vi "createEvent.vi"(8 "error in (no error)":errorcluster, 11 "Event in":refnum<class "Event.lvclass">) -> (0 "error out":errorcluster, 3 "Event out":refnum<class "Event.lvclass">)   [LabVIEW 2009, in "Events.lvlib" / "Event.lvclass"]
uses:
  Event.lvclass
  Event.lvclass/Event.ctl
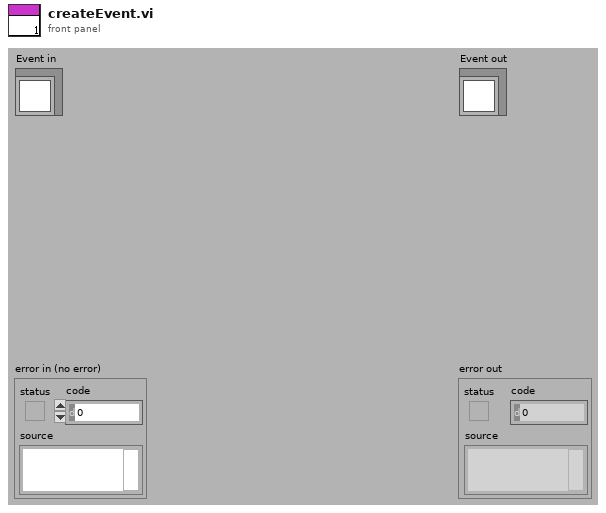
[diagram p1: front panel]
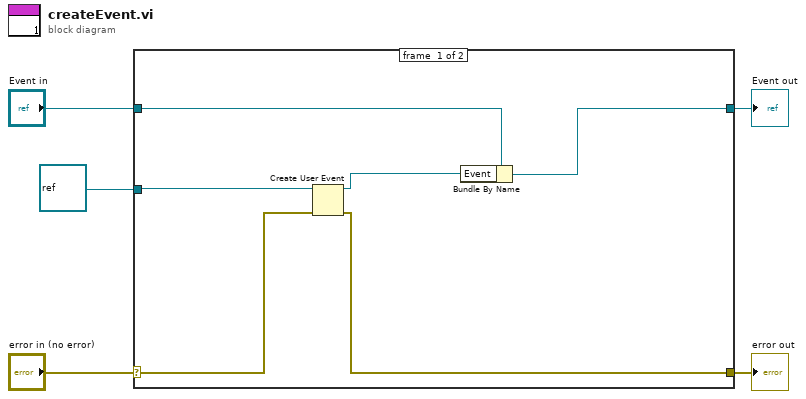
[diagram p0: block diagram]
diagram:
  n1 = case shown="No Error" "error in (no error)" {
    selector: "error in (no error)" -> [w10 w13]
    tunnel: [w9 w13] -> w4
    tunnel: [w7 w12] -> w2
    tunnel: "Event in" -> [w8 w12]
    tunnel: refnum<class> refnum ("data") -> [w11 _]
    frame #0 {
      n2 = Create User Event(user event datatype=w11, error in=w10) -> (user event=w6:refnum<user-event>, error out=w9:errorcluster)
      n3 = Bundle By Name(cluster=w8, "Event"=w6) -> (w7:refnum<class "Event.lvclass">)
    }
    frame #1 {
    }
  }
  "error out" <- w4
  "Event out" <- w2
